vi "AP_project.vi"() -> ()   [LabVIEW 2019]
uses:
  <vilib>/userDefined/High Color/IMAQdx.ctl
  <vilib>/vision/driver/IMAQdx.llb/IMAQdx Acquisition Mode.ctl
  <vilib>/vision/driver/IMAQdx.llb/IMAQdx Buffer Number Mode.ctl
  <vilib>/vision/driver/NI_Vision_Acquisition_Software.lvlib
  <vilib>/vision/NI_Vision_Development_Module.lvlib
panel:
  out "DisplayFrameRate":dbl(knob) scale=0.0..100.0 scale format="%.1f"
  in  "IMAQdx Session":T1="cam0"
  out "ProcessBufferNumber":u32
  out "ProcessFrameRate":dbl(knob) scale=0.0..100.0 scale format="%.1f"
  out "Processed Image":T2(plugin-control)
  out "# elements in queue":i32(knob) scale=0.0..250.0
  in  "Add Delay to process loop (ms)":u32
  in  "Range":cluster{"Lower value":sgl, "Upper value":sgl}={"Lower value"=50.0, "Upper value"=140.0} {"Upper value" format="%.2f"; "Lower value" format="%.2f"}
  in  "stop":bool
  out "CameraFrameRate":dbl(knob) scale=0.0..100.0 scale format="%.1f"
  out "CameraBuffer Number":u32
  out "Acquired Image":T2(plugin-control)
  out "height":dbl
  out "width":dbl
  in  "Image Path 1":path=path "C:/Program Files/National Instruments/Vision/Examples/Images/Candy1.png"
  in  "Display Index":i32
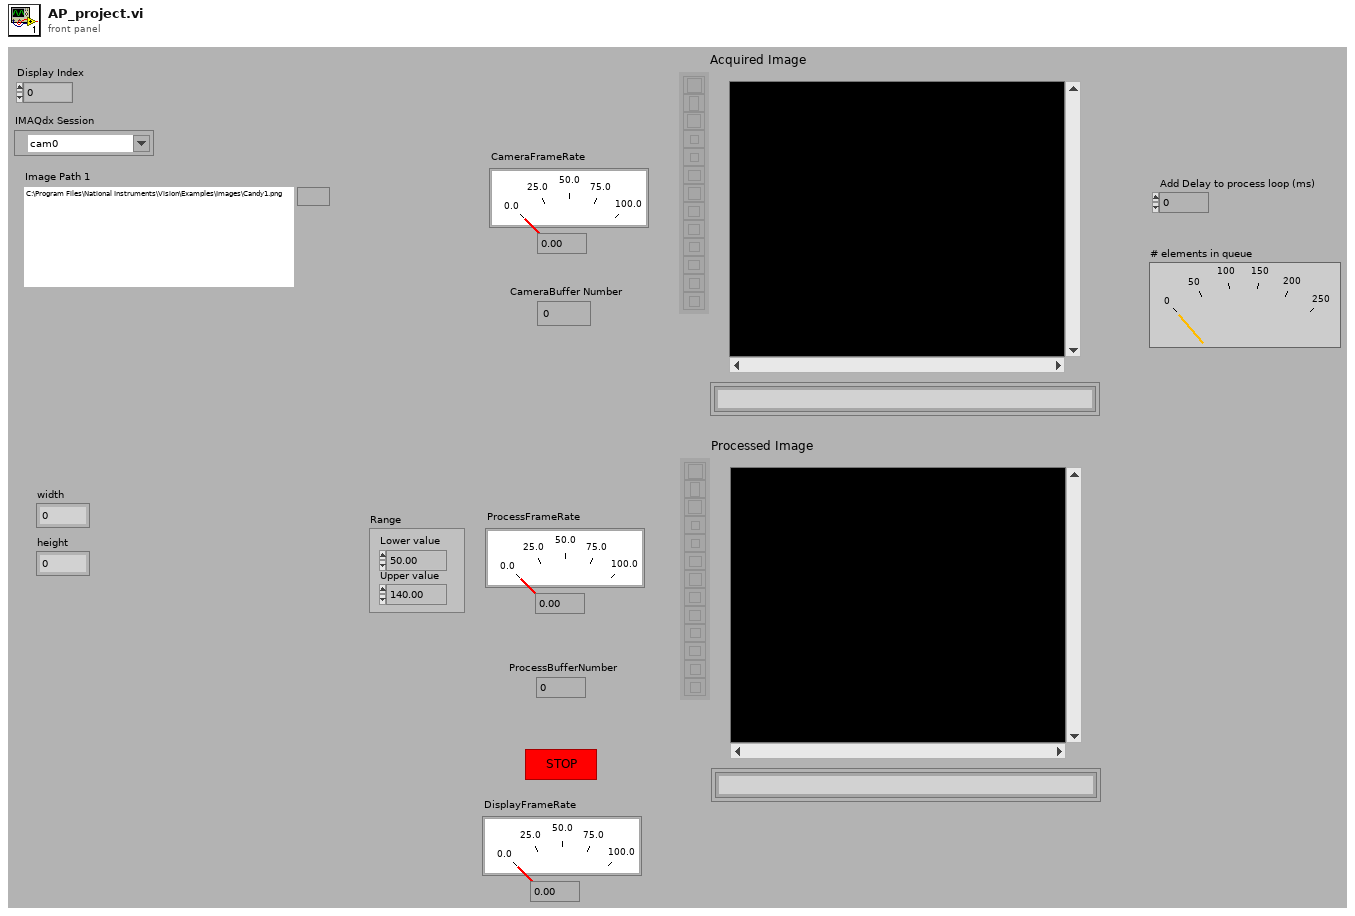
[diagram p1: front panel]
types:
  T1 = typedef "IMAQdx.ctl" = refnum<k21>
  T2 = typedef "IMAQ Image.ctl" = refnum<image>
  T3 = typedef "NI_Vision_Acquisition_Software.lvlib/IMAQdx Buffer Number Mode.ctl" = enum32{"Next", "Last", "Buffer Number", "Every", "Last New"}
  T4 = typedef "LVAllMonitorsDisplayTypeDef.ctl" = cluster{"Bounds":cluster{"Left":i16, "Top":i16, "Right":i16, "Bottom":i16}, "Depth":i16}[]
  T5 = cluster{"Bounds":cluster{"Left":i16, "Top":i16, "Right":i16, "Bottom":i16}, "Depth":i16}
  T6 = typedef "Image Type" = u32
  T7 = typedef "NI_Vision_Acquisition_Software.lvlib/IMAQdx Acquisition Mode.ctl" = enum32{"One Shot", "Continuous"}
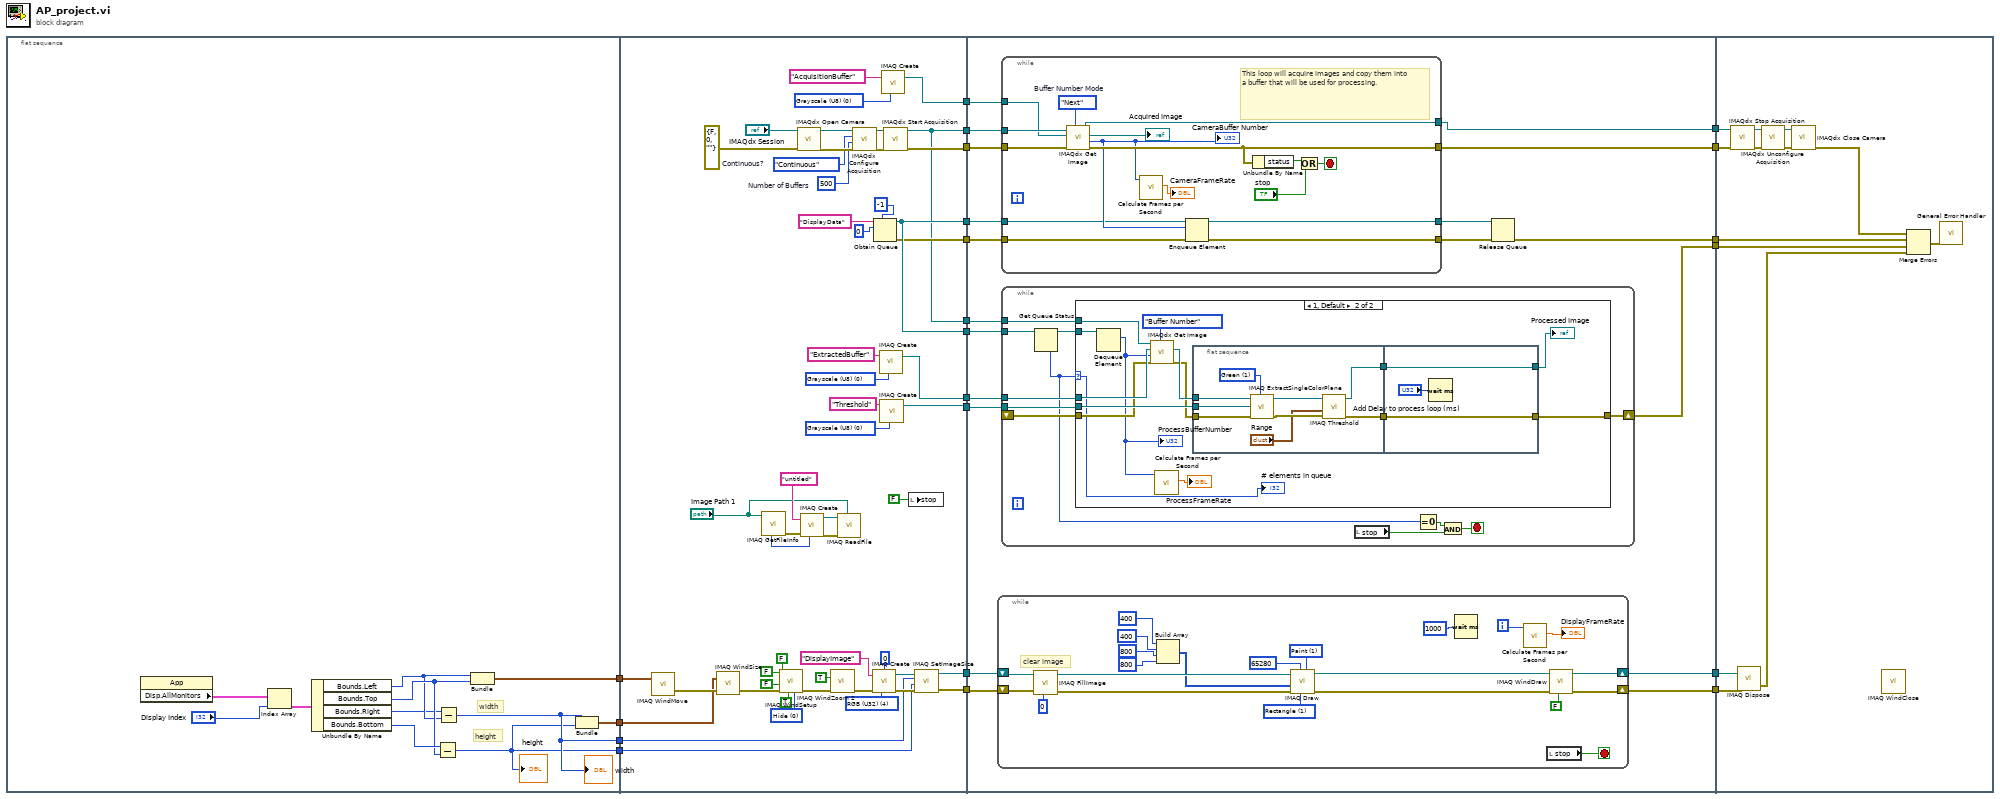
[diagram p0: block diagram]
diagram:
  n1 = flat-sequence {
    tunnel: [w25] -> w20
    tunnel: [w24] -> w19
    tunnel: [w23] -> w4
    tunnel: [w22] -> w3
    tunnel: [w41] -> w21
    tunnel: w20 -> [w81]
    tunnel: w19 -> [w79]
    tunnel: [w57] -> w18
    tunnel: [w56] -> w17
    tunnel: [w55] -> w16
    tunnel: [w54] -> w15
    tunnel: [w54] -> w14
    tunnel: [w53] -> w13
    tunnel: [w52] -> w12
    tunnel: [w51] -> w7
    tunnel: [w51] -> w6
    tunnel: [w36] -> w5
    tunnel: w4 -> [w35]
    tunnel: w3 -> [w34]
    tunnel: w21 -> [w103]
    tunnel: w18 -> [w100]
    tunnel: w17 -> [w99]
    tunnel: w16 -> [w98]
    tunnel: w15 -> [w97]
    tunnel: w14 -> [w96]
    tunnel: w13 -> [w95]
    tunnel: w12 -> [w94]
    tunnel: [w93] -> w11
    tunnel: [w92] -> w10
    tunnel: [w91] -> w9
    tunnel: [w90] -> w8
    tunnel: w7 -> [w89]
    tunnel: w6 -> [w88]
    tunnel: w5 -> [w87]
    tunnel: [w86] -> w2
    tunnel: [w85] -> w1
    tunnel: w11 -> [w192]
    tunnel: w10 -> [w191]
    tunnel: w9 -> [w186]
    tunnel: w8 -> [w185]
    tunnel: w2 -> [w183]
    tunnel: w1 -> [w182]
    frame #0 {
      # "height"
      # "width"
      n2 = property class="App"() -> ("Disp.AllMonitors"=w28:T4)  [unwired: 2 in, 2 out]
      n3 = Index Array(array=w28, index="Display Index") -> (element=w27:T5)
      n4 = Unbundle By Name(w27) -> ("Bounds.Left"=w30:i16, "Bounds.Top"=w31:i16, "Bounds.Right"=w29:i16, "Bounds.Bottom"=w32:i16)
      n5 = Subtract(x=w32, y=w31) -> (x-y=w22:i16)
      "height" <- w22
      n6 = Subtract(x=w29, y=w30) -> (x-y=w23:i16)
      "width" <- w23
      n7 = Bundle("Left"=w30, "Top"=w31) -> (w24:cluster{"Left":i16, "Top":i16})  [unwired: 1 in]
      n8 = Bundle(w23, w22) -> (w25:cluster{i16, i16})  [unwired: 1 in]
    }
    frame #1 {
      w37 = T6 4 items=["Grayscale (U8)", "Grayscale (I16)", "Grayscale (SGL)", "Complex (CSG)", "RGB (U32)", "HSL (U32)", "RGB (U64)"] ("Image Type")
      w67 = T6 0 items=["Grayscale (U8)", "Grayscale (I16)", "Grayscale (SGL)", "Complex (CSG)", "RGB (U32)", "HSL (U32)", "RGB (U64)"] ("Image Type")
      w65 = T6 0 items=["Grayscale (U8)", "Grayscale (I16)", "Grayscale (SGL)", "Complex (CSG)", "RGB (U32)", "HSL (U32)", "RGB (U64)"] ("Image Type")
      w58 = T6 0 items=["Grayscale (U8)", "Grayscale (I16)", "Grayscale (SGL)", "Complex (CSG)", "RGB (U32)", "HSL (U32)", "RGB (U64)"] ("Image Type")
      w64 = u32 500  # Number of Buffers
      w63 = IMAQdx_Acquisition_Mode."Continuous"  # Continuous?
      w78 = 0 items=["Hide", "Show", "No change"] ("Scrollbars (No change)")
      n9 = call "IMAQ WindMove"("Coordinates (screen)"=w79) -> ("error out"=w83:errorcluster)  [unwired: 4 in, 1 out]
      n10 = call "IMAQ WindSize"("error in (no error)"=w83, "Width & Height"=w81) -> ("error out"=w84:errorcluster)  [unwired: 4 in, 2 out]
      n11 = call "IMAQ GetFileInfo"("File Path"="Image Path 1") -> ("error out"=w46:errorcluster, "Image Type"=w48:T6)  [unwired: 4 in, 5 out]
      n12 = call "IMAQ WindSetup"("Scrollbars (No change)"=w78, "Window is floating? (No)"=TRUE, "error in (no error)"=w84, "Window has title bar? (Yes)"=FALSE, "Window can close? (Yes)"=FALSE, "Window can grow? (Yes)"=FALSE) -> ("error out"=w82:errorcluster)  [unwired: 5 in]
      n13 = call <vilib>:"IMAQdx Open Camera.vi"("error in"=errorcluster {"status"=FALSE, "code"=0, "source"=""}, "Session In"="IMAQdx Session") -> ("error out"=w72:errorcluster, "Session Out"=w73:T1)  [unwired: 8 in]
      n14 = call "IMAQ Create"("Image Name"="untitled", "Image Type"=w48, "error in (no error)"=w46) -> ("New Image"=w44:T2, "error out"=w45:errorcluster)  [unwired: 2 in]
      n15 = call "IMAQ WindZoom 2"("error in (no error)"=w82, "Zoom to Fit? (False)"=TRUE ("Zoom to Fit? (T)")) -> ("error out"=w40:errorcluster)  [unwired: 6 in, 3 out]
      n16 = call "IMAQ ReadFile"("File Path"="Image Path 1", "error in (no error)"=w45, "Image"=w44) -> ()  [unwired: 4 in, 5 out]
      n17 = call <vilib>:"IMAQdx Configure Acquisition.vi"("error in"=w72, "Number of Buffers"=w64, "Continuous?"=w63, "Session In"=w73) -> ("error out"=w71:errorcluster, "Session Out"=w69:T1)  [unwired: 6 in]
      n18 = call "IMAQ Create"("Border Size"=0, "Image Name"="DisplayImage", "Image Type"=w37, "error in (no error)"=w40) -> ("New Image"=w42:T2, "error out"=w43:errorcluster)  [unwired: 1 in]
      n19 = Obtain Queue(max queue size (-1, unlimited)=-1, name (unnamed)="DisplayData", element data type=u32 0) -> (queue out=w54:refnum<queue>, error out=w53:errorcluster)  [unwired: 2 in, 1 out]
      n20 = call "IMAQ Create"("Image Name"="ExtractedBuffer", "Image Type"=w67) -> ("New Image"=w57:T2)  [unwired: 3 in, 1 out]
      n21 = call "IMAQ Create"("Image Name"="Threshold", "Image Type"=w65) -> ("New Image"=w56:T2)  [unwired: 3 in, 1 out]
      n22 = call "IMAQ Create"("Image Name"="AcquisitionBuffer", "Image Type"=w58) -> ("New Image"=w52:T2)  [unwired: 3 in, 1 out]
      n23 = call <vilib>:"IMAQdx Start Acquisition.vi"("error in"=w71, "Session In"=w69) -> ("error out"=w55:errorcluster, "Session Out"=w51:T1)  [unwired: 8 in]
      n24 = local write "stop"(FALSE ("stop")) -> ()
      n25 = call "IMAQ SetImageSize"("error in (no error)"=w43, "Y Resolution"=w34, "X Resolution"=w35, "Image"=w42) -> ("error out"=w41:errorcluster, "Image Out"=w36:T2)  [unwired: 1 in]
    }
    frame #2 {
      n26 = while {
        shift-right: [w174] -> w86
        shift-left: w87 -> [w178]
        shift-right: [w173] -> w85
        shift-left: w103 -> [w177]
        i -> [w172]
        stop <- w179 stop-if-true
        w167 = u16 1 items=["Frame", "Paint", "Invert Frame", "Invert Paint"] ("Draw Mode")
        w166 = u16 1 items=["Line", "Rectangle", "Oval"] ("Shape to draw")
        # "clear image"
        n27 = call "IMAQ FillImage"("Color Pixel Value"=0, "error in (no error)"=w177, "Image"=w178) -> ("error out"=w168:errorcluster, "Image Out"=w164:T2)  [unwired: 7 in]
        n28 = Build Array(400, 400, 800, 800) -> (w163:i32[])
        n29 = call "IMAQ Draw"("Draw Mode"=w167, "Shape to draw"=w166, "Pixel Color"=65280, "error in (no error)"=w168, "Coordinates"=w163, "Image Src"=w164) -> ("error out"=w169:errorcluster, "Image Dst Out"=w170:T2)  [unwired: 4 in]
        n30 = Wait (ms)(milliseconds to wait=u32 1000) -> ()  [unwired: 1 out]
        n31 = call <vilib>:"Calculate Frames per Second.vi"("Buffer Number"=w172) -> ("Processed Frames/s"=→"DisplayFrameRate":dbl)  [unwired: 8 in, 2 out]
        n32 = local read "stop"() -> (w179:bool)
        n33 = call "IMAQ WindDraw"("Resize to Image Size? (Y)"=FALSE, "error in (no error)"=w169, "Image"=w170) -> ("error out"=w173:errorcluster, "Image Out (duplicate)"=w174:T2)  [unwired: 7 in]
      }
      n34 = while {
        tunnel: [w150] -> w91
        tunnel: [w155] -> w90
        tunnel: [w154] -> w101
        tunnel: [w153] -> w102
        tunnel: w98 -> [w147]
        tunnel: w96 -> [w145]
        tunnel: w95 -> [w144]
        tunnel: w94 -> [w143]
        tunnel: w89 -> [w146]
        stop <- w158 stop-if-true
        w152 = IMAQdx_Buffer_Number_Mode."Next"  # Buffer Number Mode
        # "This loop will acquire images and copy them into a buffer that will be used for processing."
        n35 = call <vilib>:"IMAQdx Get Image.vi"("Buffer Number Mode (Next)"=w152, "error in"=w147, "Image In"=w143, "Session In"=w146) -> ("error out"=w150:errorcluster, "Buffer Number Out"=w148:u32, "Image Out"=→"Acquired Image":T2, "Session Out"=w155:T1)  [unwired: 4 in]
        "CameraBuffer Number" <- w148
        n36 = call <vilib>:"Calculate Frames per Second.vi"("Buffer Number"=w148) -> ("Processed Frames/s"=→"CameraFrameRate":dbl)  [unwired: 8 in, 2 out]
        n37 = Enqueue Element(queue=w145, element=w148, error in (no error)=w144) -> (queue out=w154:refnum<queue>, error out=w153:errorcluster)  [unwired: 1 in, 1 out]
        n38 = Unbundle By Name(w150) -> ("status"=w157:bool)
        n39 = Or(x=w157, y="stop") -> (x .or. y?=w158:bool)
      }
      n40 = while {
        shift-right: [w112] -> w92
        shift-left: _ -> [w113]
        tunnel: w100 -> [w111]
        tunnel: w99 -> [w110]
        tunnel: w88 -> [w109]
        tunnel: w97 -> [w108]
        stop <- w107 stop-if-true
        n41 = Get Queue Status(queue=w108) -> (queue out=w114:refnum<queue>, # elements in queue=w104:i32)  [unwired: 2 in, 6 out]
        n42 = case shown="1, Default" w104 {
          selector: w104 -> [_ w120]
          tunnel: w114 -> [_ w130]
          tunnel: w111 -> [_ w124]
          tunnel: w113 -> [w115 w122]
          tunnel: w110 -> [_ w129]
          tunnel: [w115 w128] -> w112
          tunnel: w109 -> [_ w126]
          frame 0 {
          }
          frame 1, Default {
            n43 = Dequeue Element(queue=w130) -> (element=w117:u32)  [unwired: 2 in, 3 out]
            "ProcessBufferNumber" <- w117
            n44 = call <vilib>:"IMAQdx Get Image.vi"("Buffer Number Mode (Next)"=IMAQdx_Buffer_Number_Mode."Buffer Number", "error in"=w122, "Buffer Number In"=w117, "Image In"=w124, "Session In"=w126) -> ("error out"=w121:errorcluster, "Image Out"=w123:T2)  [unwired: 3 in, 2 out]
            n45 = call <vilib>:"Calculate Frames per Second.vi"("Buffer Number"=w117) -> ("Processed Frames/s"=→"ProcessFrameRate":dbl)  [unwired: 8 in, 2 out]
            n46 = flat-sequence {
              tunnel: w129 -> [w139]
              tunnel: w123 -> [w132]
              tunnel: w121 -> [w131]
              tunnel: [w136] -> w119
              tunnel: [w134] -> w118
              tunnel: [w141] -> w127
              tunnel: [w142] -> w128
              tunnel: w119 -> [w142]
              tunnel: w118 -> [w141]
              frame #0 {
                w138 = 1 items=["Red", "Green", "Blue", "Hue", "Saturation", "Luminance", "Value", "Intensity"] ("Color Plane")
                n47 = call "IMAQ ExtractSingleColorPlane"("Color Plane"=w138, "error in (no error)"=w131, "Image Dst"=w139, "Image Src"=w132) -> ("error out"=w137:errorcluster, "Image Dst Out"=w135:T2)  [unwired: 6 in]
                n48 = call "IMAQ Threshold"("error in (no error)"=w137, "Range"="Range", "Image Src"=w135) -> ("error out"=w136:errorcluster, "Image Dst Out"=w134:T2)  [unwired: 7 in]
              }
              frame #1 {
                n49 = Wait (ms)(milliseconds to wait="Add Delay to process loop (ms)") -> ()  [unwired: 1 out]
              }
            }
            "Processed Image" <- w127
            "# elements in queue" <- w120
          }
        }
        n50 = local read "stop"() -> (w106:bool)
        n51 = Equal To 0?(x=w104) -> (x = 0?=w105:bool)
        n52 = And(x=w105, y=w106) -> (x .and. y?=w107:bool)
      }
      n53 = Release Queue(queue=w101, error in (no error)=w102) -> (error out=w93:errorcluster)  [unwired: 1 in, 2 out]
    }
    frame #3 {
      n54 = call <vilib>:"IMAQdx Stop Acquisition.vi"("error in"=w186, "Session In"=w185) -> ("error out"=w187:errorcluster, "Session Out"=w188:T1)  [unwired: 8 in]
      n55 = call "IMAQ Dispose"("Image"=w183, "error in (no error)"=w182) -> ("error out"=w181:errorcluster)  [unwired: 4 in]
      n56 = call <vilib>:"IMAQdx Unconfigure Acquisition.vi"("error in"=w187, "Session In"=w188) -> ("error out"=w190:errorcluster, "Session Out"=w189:T1)  [unwired: 8 in]
      n57 = call <vilib>:"IMAQdx Close Camera.vi"("error in"=w190, "Session In"=w189) -> ("error out"=w184:errorcluster)  [unwired: 9 in]
      n58 = call "IMAQ WindClose"() -> ()  [unwired: 6 in, 1 out]
      n59 = Merge Errors(w184, w192, w191, w181) -> (w193:errorcluster)
      n60 = call <vilib>:"General Error Handler.vi"("error in (no error)"=w193) -> ()  [unwired: 10 in, 5 out]
    }
  }
